vi "Create Shared Resources.vi"(8 "error in":errorcluster, 10 "custom device ref":T1=18446744073709551615 format="%.0x", 11 "shared resources factory in":refnum<class "Shared Resources Factory.lvclass">) -> (0 "error out":errorcluster, 2 "shared resources":refnum<class "Shared Resources.lvclass">, 3 "shared resources factory out":refnum<class "Shared Resources Factory.lvclass">)   [LabVIEW 2020, in "Ballard ARINC 429 Engine.lvlib" / "Implementation.lvlib" / "Shared Resources Factory.lvclass"]
uses:
  Shared Resources Factory.lvclass
  <vilib>/NI VeriStand/Custom Device API/Custom Device Item Ref.ctl
  Interfaces/Shared Resources/Shared Resources.lvclass
  Shared Resources/Shared Resources.lvclass
  C:/Git/niveristand-ballard-arinc429-custom-device/Source/Custom Device Support/Engine/Interfaces/Shared Resources/Shared Resources.lvclass
  Scripting/Ballard/Ballard ARINC 429 Scripting.lvlib
  <vilib>/NI VeriStand/Custom Device API/Custom Device API.lvlib
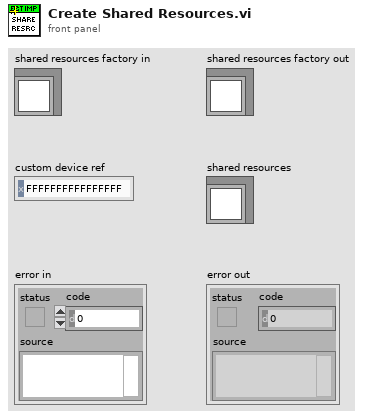
[diagram p1: front panel]
types:
  T1 = typedef "Custom Device API.lvlib/Custom Device Item Ref.ctl" = u64
  T2 = typedef "Device Parameters.ctl" = cluster{"initialization method":T3, "card number":i32, "PXI slot number":i32, "core number":i32}
  T3 = typedef "Initialization Method.ctl" = enum16{"PXI Slot Number", "Card Number"}
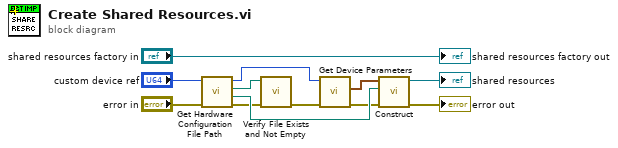
[diagram p0: block diagram]
diagram:
  n1 = call "Get Hardware Configuration File Path.vi"("error in"="error in", "custom device ref"="custom device ref") -> ("error out"=w7:errorcluster, "RTDestination"=w10:path, "path"=w8:path, "custom device ref out"=w1:T1)  [unwired: 6 in]
  n2 = call "Verify File Exists and Not Empty.vi"("error in"=w7, "path"=w8) -> ("error out"=w5:errorcluster)  [unwired: 9 in]
  n3 = call "Get Device Parameters.vi"("error in"=w5, "Ballard ARINC 429 custom device in"=w1) -> ("error out"=w4:errorcluster, "device parameters"=w11:T2)  [unwired: 7 in, 1 out]
  n4 = call "Construct.vi"("error in"=w4, "hardware configuration file on target"=w10, "device parameters"=w11) -> ("error out"=→"error out":errorcluster, "Ballard ARINC-429 shared resources out"=→"shared resources":refnum<class "Shared Resources.lvclass">)  [unwired: 7 in]
  "shared resources factory out" <- "shared resources factory in"
